vi "Initialize.vi"(8 "error in":errorcluster, 10 "Device":string) -> (0 "error out":errorcluster, 3 "Function Generator out":refnum<class "Function Generator.lvclass">)   [LabVIEW 2018, in "Function Generator.lvlib" / "Function Generator.lvclass"]
uses:
  Function Generator.lvclass
  Function Generator.lvclass/Function Generator.ctl
  builds/Configuration.lvlibp/Configuration.lvclass
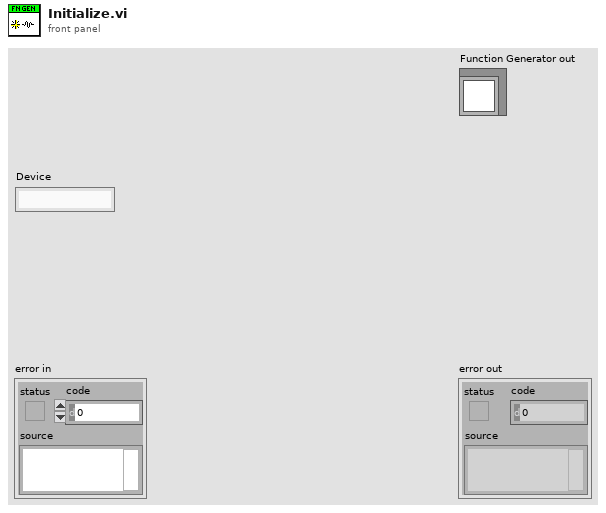
[diagram p1: front panel]
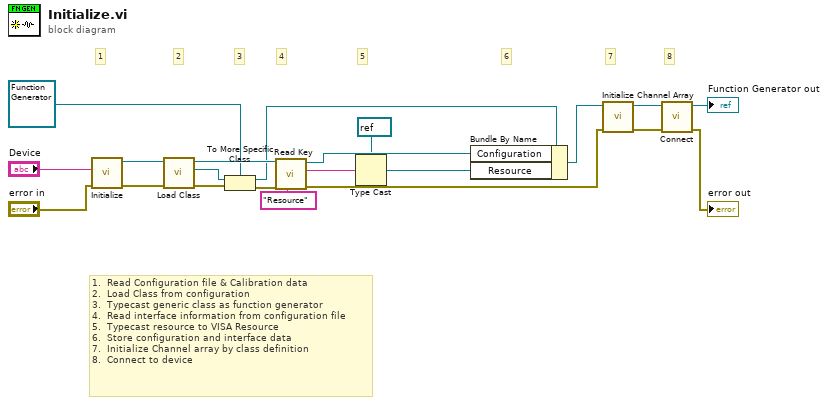
[diagram p0: block diagram]
diagram:
  # "8"
  # "7"
  # "1.  Read Configuration file & Calibration data\n2.  Load Class from configuration\n3.  Typecast generic class as function generator\n4.  Read interface information from configuration file\n5.  Typecast resource to VISA Resource\n6.  Store configuration and interface data\n7.  Initialize Channel array by class definition\n8.  Connect to device"
  # "6"
  # "5"
  # "4"
  # "3"
  # "2"
  # "1"
  n1 = call "Initialize.vi"("error in"="error in", "Device"="Device") -> ("error out"=w19:errorcluster, "Configuration out"=w18:refnum<class "Configuration.lvclass">)  [unwired: 8 in]
  n2 = call "Load Class.vi"("error in"=w19, "Configuration in"=w18) -> ("error out"=w15:errorcluster, "Class out"=w14:refnum<class>, "Configuration out"=w17:refnum<class "Configuration.lvclass">)  [unwired: 7 in]
  n3 = To More Specific Class(target class=refnum<class "Function Generator.lvclass"> refnum ("Function Generator in"), reference=w14, error in=w15) -> (specific class reference=w11:refnum<class "Function Generator.lvclass">, error out=w16:errorcluster)
  n4 = call "Read Key.vi"("Key:"="Resource", "error in"=w16, "Configuration in"=w17) -> ("error out"=w5:errorcluster, "Value"=w9:string, "Configuration out"=w10:refnum<class "Configuration.lvclass">)  [unwired: 6 in]
  n5 = Type Cast(type=refnum<visa-resource-name> refnum ("Resource"), x=w9) -> (*(type *) &x=w7:refnum<visa-resource-name>)
  n6 = Bundle By Name(cluster=w11, "Configuration"=w10, "Resource"=w7) -> (w6:refnum<class "Function Generator.lvclass">)
  n7 = call "Initialize Channel Array.vi"("error in"=w5, "Function Generator in"=w6) -> ("error out"=w3:errorcluster, "Function Generator out"=w4:refnum<class "Function Generator.lvclass">)  [unwired: 8 in]
  n8 = call-dynamic "Connect.vi"("error in (no error)"=w3, "Function Generator in"=w4) -> ("error out"=→"error out":errorcluster, "Function Generator out"=→"Function Generator out":refnum<class "Function Generator.lvclass">)  [unwired: 8 in]
